vi "ByteArrayToNumber.vi"(11 "In Array":u8[](array[numeric])) -> (3 "Out Number":u32)   [LabVIEW 2019]
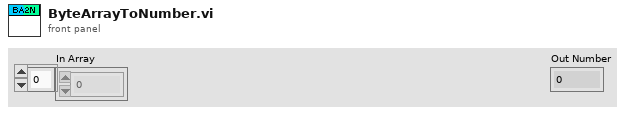
[diagram p1: front panel]
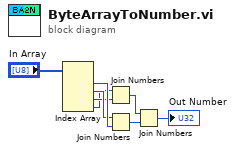
[diagram p0: block diagram]
diagram:
  n1 = Index Array(array="In Array") -> (element #1=w5:u8, element #2=w4:u8, element #3=w3:u8, element #4=w2:u8)  [unwired: 4 in]
  n2 = Join Numbers(hi=w2, lo=w3) -> ((hi.lo)=w7:u16)
  n3 = Join Numbers(hi=w4, lo=w5) -> ((hi.lo)=w6:u16)
  n4 = Join Numbers(hi=w7, lo=w6) -> ((hi.lo)=→"Out Number":u32)
